vi "EvalTimes.vi"(4 "Total_Delta_In":i32, 5 "Max_In":i32, 6 "Iteration":i32, 7 "Init_Time":i32) -> (0 "Total_Delta_Out":i32, 1 "Mean":dbl, 2 "Max_Out":i32, 3 "Delta":i32)   [LabVIEW 2015]
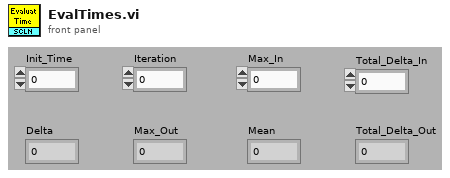
[diagram p1: front panel]
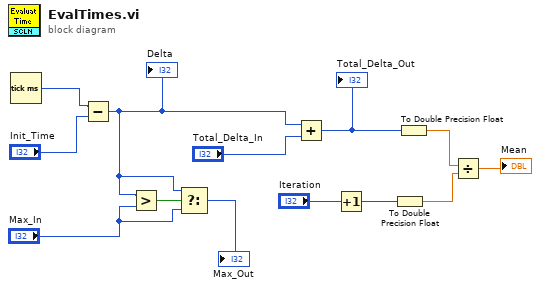
[diagram p0: block diagram]
diagram:
  n1 = Tick Count (ms)() -> (millisecond timer value=w13:u32)
  n2 = Subtract(x=w13, y="Init_Time") -> (x-y=w7:u32)
  "Delta" <- w7
  n3 = Greater?(x=w7, y="Max_In") -> (0:w11:bool)
  n4 = Select(t=w7, s=w11, f="Max_In") -> (s? t:f=→"Max_Out":u32)
  n5 = Add(x=w7, y="Total_Delta_In") -> (x+y=w6:u32)
  "Total_Delta_Out" <- w6
  n6 = Increment(x="Iteration") -> (x+1=w1:i32)
  n7 = To Double Precision Float(number=w1) -> (double precision float=w3:dbl)
  n8 = To Double Precision Float(number=w6) -> (double precision float=w4:dbl)
  n9 = Divide(x=w4, y=w3) -> (x/y=→"Mean":dbl)
